vi "Phase detector test.vi"() -> ()   [LabVIEW 2016]
panel:
  in  "Stop Button":bool
  in  "Guess angle":dbl(slide)=-2.87556 scale=-7.0..7.0
  in  "Initial parameters":dbl[](array[numeric])=[188.484, 0.01, 0.00126452, 2.4, 1.1376494443646765, -0.8104040332703796]
  out "Circle fit":cluster{"Array":dbl[], "Array":dbl[]}[](graph)
  out "Fit":cluster{"X":dbl[], "best nonlinear fit":dbl[]}[](graph)
  in  "Z":cdb[](array[numeric])
  in  "Z":cdb[](array[numeric])
  in  "X":dbl[](array[numeric])
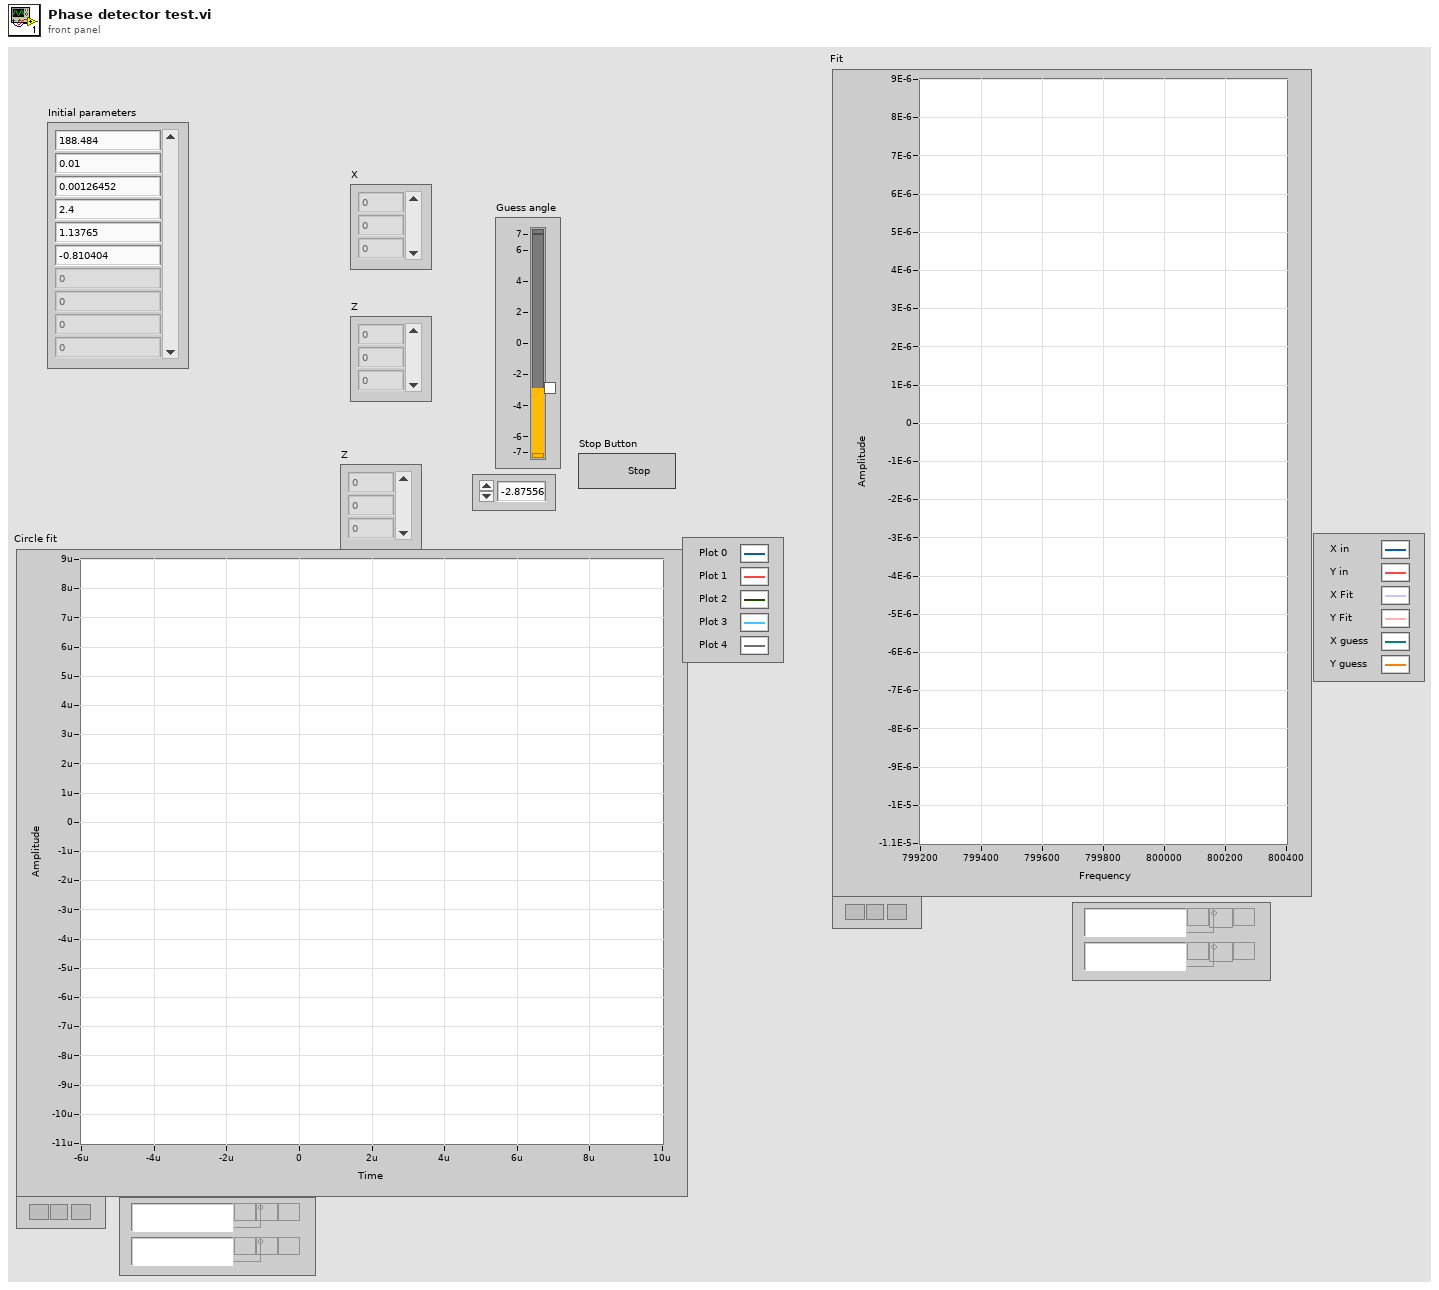
[diagram p1: front panel]
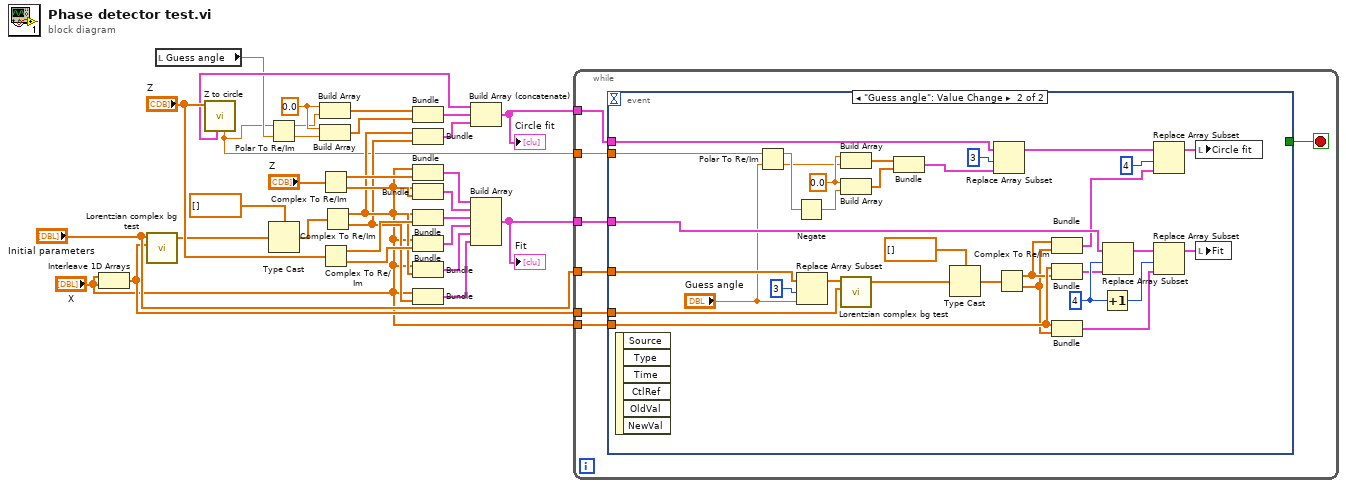
[diagram p0: block diagram]
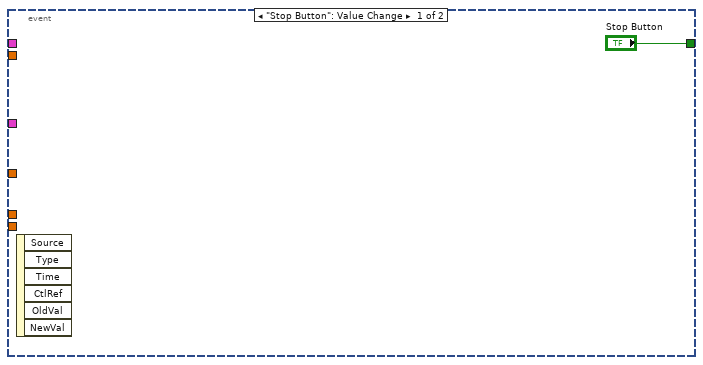
[diagram p2: hidden frame]
diagram:
  w14 = 0.0
  n1 = Interleave 1D Arrays("X", "X") -> (w9:dbl[])
  n2 = call "Lorentzian complex bg test.vi"("X"=w9, "a"="Initial parameters") -> ("f(X,a)"=w20:dbl[])  [unwired: 2 in, 2 out]
  n3 = local read "Guess angle"() -> (w2:dbl)
  n4 = call "Z to circle.vi"("Z"="Z") -> ("r"=w1:dbl, "Circle fit"=w22:cluster{"Array":dbl[], "Array":dbl[]}[])  [unwired: 4 in, 5 out]
  n5 = Polar To Re/Im(2:w2, 3:w1) -> (0:w11:dbl, 1:w13:dbl)
  n6 = Type Cast(type=cdb[] [], x=w20) -> (*(type *) &x=w19:cdb[])
  n7 = Build Array(w14, w13) -> (w15:dbl[])
  n8 = Build Array(w14, w11) -> (w16:dbl[])
  n9 = Complex To Re/Im(x + iy="Z") -> (x=w31:dbl[], y=w28:dbl[])
  n10 = Complex To Re/Im(x + iy="Z") -> (x=w29:dbl[], y=w30:dbl[])
  n11 = Complex To Re/Im(x + iy=w19) -> (x=w7:dbl[], y=w6:dbl[])
  n12 = Bundle(w15, w16) -> (w12:cluster{dbl[], dbl[]})  [unwired: 1 in]
  n13 = Bundle(w7, w6) -> (w8:cluster{dbl[], dbl[]})  [unwired: 1 in]
  n14 = Bundle("X"="X", w31) -> (w27:cluster{"X":dbl[], dbl[]})  [unwired: 1 in]
  n15 = Bundle("X"="X", w28) -> (w26:cluster{"X":dbl[], dbl[]})  [unwired: 1 in]
  n16 = Bundle("X"="X", w29) -> (w25:cluster{"X":dbl[], dbl[]})  [unwired: 1 in]
  n17 = Bundle("X"="X", w30) -> (w24:cluster{"X":dbl[], dbl[]})  [unwired: 1 in]
  n18 = Bundle("X"="X", w7) -> (w17:cluster{"X":dbl[], dbl[]})  [unwired: 1 in]
  n19 = Bundle("X"="X", w6) -> (w18:cluster{"X":dbl[], dbl[]})  [unwired: 1 in]
  n20 = Build Array (concatenate)(w22, w12, w8) -> (w3:cluster{"Array":dbl[], "Array":dbl[]}[])
  "Circle fit" <- w3
  n21 = Build Array(w27, w26, w25, w24, w17, w18) -> (w4:cluster{"X":dbl[], dbl[]}[])
  "Fit" <- w4
  n22 = while {
    tunnel: "Initial parameters" -> [w38]
    tunnel: w9 -> [w37]
    tunnel: "X" -> [w36]
    tunnel: w4 -> [w35]
    tunnel: w3 -> [w34]
    tunnel: w1 -> [w33]
    stop <- w39 stop-if-true
    n23 = event shown="[1] \"Guess angle\": Value Change" {
      selector: _ -> [_ _]
      dyn-events: _ -> [_ _]
      timeout: _ -> [_ _]
      tunnel: ["Stop Button" _] -> w39
      tunnel: w38 -> [_ w72]
      tunnel: w37 -> [_ w69]
      tunnel: w36 -> [_ w66]
      tunnel: w35 -> [_ w64]
      tunnel: w34 -> [_ w58]
      tunnel: w33 -> [_ w50]
      event "Stop Button": Value Change {
        n24 = event-data() -> ()  [unwired: 1 in, 6 out]
      }
      event "Guess angle": Value Change {
        w51 = 0.0
        w63 = 4 ("index")
        n25 = event-data() -> ()  [unwired: 1 in, 6 out]
        n26 = Polar To Re/Im(2:"Guess angle", 3:w50) -> (0:w42:dbl, 1:w43:dbl)
        n27 = Negate(x=w43) -> (-x=w41:dbl)
        n28 = Replace Array Subset(array=w72, new element="Guess angle", index=3) -> (w70:dbl[])
        n29 = Build Array(w51, w42) -> (w47:dbl[])
        n30 = Build Array(w51, w41) -> (w46:dbl[])
        n31 = call "Lorentzian complex bg test.vi"("X"=w69, "a"=w70) -> ("f(X,a)"=w65:dbl[])  [unwired: 2 in, 2 out]
        n32 = Bundle(w47, w46) -> (w45:cluster{dbl[], dbl[]})  [unwired: 1 in]
        n33 = Type Cast(type=cdb[] [], x=w65) -> (*(type *) &x=w67:cdb[])
        n34 = Replace Array Subset(array=w58, new element=w45, index=3) -> (w48:cluster{"Array":dbl[], "Array":dbl[]}[])
        n35 = Complex To Re/Im(x + iy=w67) -> (x=w57:dbl[], y=w56:dbl[])
        n36 = Bundle(w57, w56) -> (w55:cluster{dbl[], dbl[]})  [unwired: 1 in]
        n37 = Bundle("X"=w66, w57) -> (w60:cluster{"X":dbl[], dbl[]})  [unwired: 1 in]
        n38 = Bundle("X"=w66, w56) -> (w59:cluster{"X":dbl[], dbl[]})  [unwired: 1 in]
        n39 = Increment(x=w63) -> (x+1=w62:i32)
        n40 = Replace Array Subset(array=w64, new element=w60, index=w63) -> (w61:cluster{"X":dbl[], dbl[]}[])
        n41 = Replace Array Subset(array=w48, new element=w55, index=4) -> (w53:cluster{"Array":dbl[], "Array":dbl[]}[])
        n42 = Replace Array Subset(array=w61, new element=w59, index=w62) -> (w52:cluster{"X":dbl[], dbl[]}[])
        n43 = local write "Circle fit"(w53) -> ()
        n44 = local write "Fit"(w52) -> ()
      }
    }
  }
